vi "makeResult.vi"(8 "error in (no error)":errorcluster, 11 "TextTestRunner in":refnum<class "TestRunner.lvclass">) -> (0 "error out":errorcluster, 2 "TestResult":refnum<class "TestResult.lvclass">, 3 "TextTestRunner out":refnum<class "TestRunner.lvclass">)   [LabVIEW 2011, in "TestRunner.lvclass"]
uses:
  TestRunner.lvclass
  TestResult/TestResult.lvclass
panel:
  # "JKI VI Tester for LabVIEW\nhttp://jkisoft.com/vi-tester\nCopyright (C) 2007-2009, JKI <info@jkisoft.com>\nALL RIGHTS RESERVED"
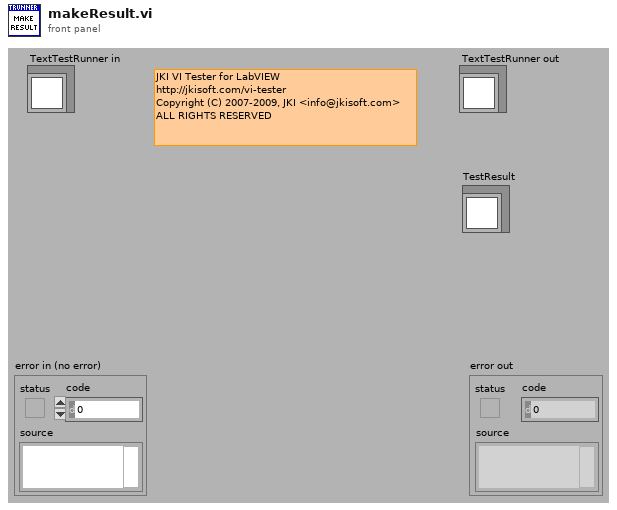
[diagram p1: front panel]
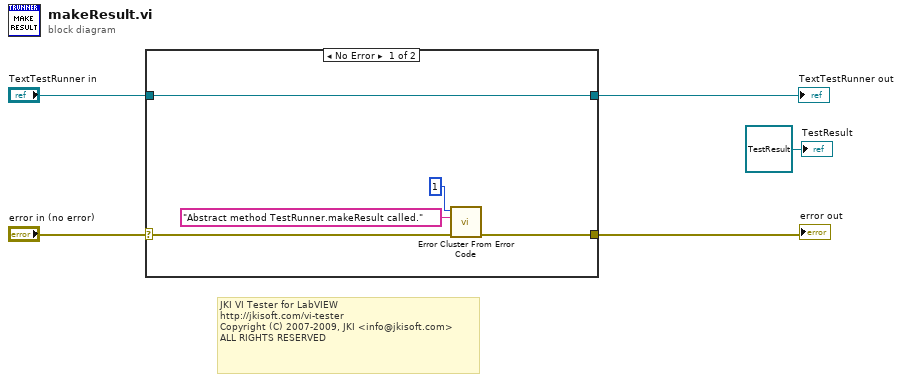
[diagram p0: block diagram]
diagram:
  # "JKI VI Tester for LabVIEW\nhttp://jkisoft.com/vi-tester\nCopyright (C) 2007-2009, JKI <info@jkisoft.com>\nALL RIGHTS RESERVED"
  n1 = case shown="No Error" "error in (no error)" {
    selector: "error in (no error)" -> [w9 w12]
    tunnel: [w8 w12] -> w4
    tunnel: [w10 w11] -> w2
    tunnel: "TextTestRunner in" -> [w10 w11]
    frame No Error {
      n2 = call <vilib>:"Error Cluster From Error Code.vi"("error in (no error)"=w9, "error message (\"\")"="Abstract method TestRunner.makeResult called." ("error message (\"\")"), "error code (0)"=1) -> ("error out"=w8:errorcluster)  [unwired: 6 in]
    }
    frame Error {
    }
  }
  "error out" <- w4
  "TextTestRunner out" <- w2
  "TestResult" <- refnum<class "TestResult.lvclass"> refnum ("TestResult")
